vi "DrawGameOver.vi"(8 "error in (no error)":errorcluster, 11 "Game in":refnum<class "Game.lvclass">) -> (0 "error out":errorcluster, 3 "Game out":refnum<class "Game.lvclass">)   [LabVIEW 2019, in "RT_Game.lvlib" / "Game.lvclass"]
uses:
  Game.lvclass
  Color.ctl
  Coordinate.ctl
  Game.lvclass/Game.ctl
  RT_Game.lvlib
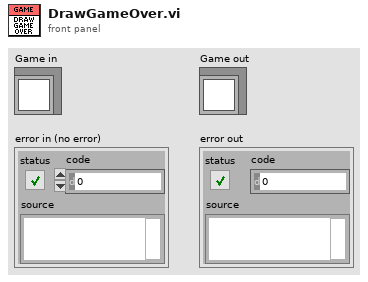
[diagram p1: front panel]
types:
  T1 = typedef "RT_Game.lvlib/Game.lvclass/Coordinate.ctl" = cluster{"x":dbl, "y":dbl}
  T2 = typedef "RT_Game.lvlib/Color.ctl" = fxp<+,3,3>
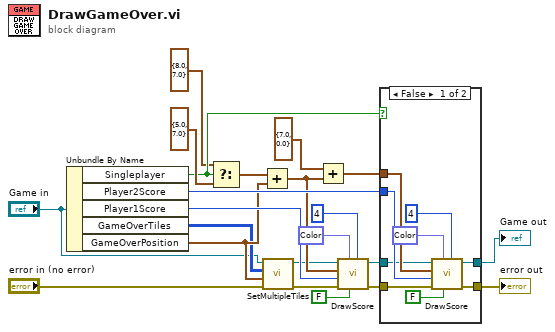
[diagram p0: block diagram]
diagram:
  n1 = Unbundle By Name("Game in") -> ("Singleplayer"=w2:bool, "Player2Score"=w22:i32, "Player1Score"=w14:i32, "GameOverTiles"=w7:u32[][], "GameOverPosition"=w12:T1)
  n2 = Select(t=T1 {"x"=8.0, "y"=7.0} ("f"), s=w2, f=T1 {"x"=5.0, "y"=7.0} ("x")) -> (s? t:f=w3:T1)
  n3 = Add(x=w3, y=w12) -> (x+y=w20:T1)
  n4 = call "SetMultipleTiles.vi"("error in (no error)"="error in (no error)", "Position"=w12, "TileCodes"=w7, "Game in"="Game in") -> ("error out"=w5:errorcluster, "Game out"=w9:refnum<class "Game.lvclass">)  [unwired: 6 in]
  n5 = Add(x=T1 {"x"=7.0, "y"=0.0}, y=w20) -> (x+y=w19:T1)
  n6 = call "DrawScore.vi"("Digits"=4, "AutoWidth?"=FALSE, "Color"=T2 1.0, "error in (no error)"=w5, "score"=w14, "position"=w20, "Pong in"=w9) -> ("error out"=w8:errorcluster, "Pong out"=w17:refnum<class "Game.lvclass">)  [unwired: 3 in]
  n7 = case shown="False" w2 {
    tunnel: w22 -> [w28 _]
    tunnel: w19 -> [w27 _]
    tunnel: [w26 w33] -> w18
    tunnel: w17 -> [w25 w33]
    tunnel: [w24 w32] -> w16
    tunnel: w8 -> [w23 w32]
    frame False {
      n8 = call "DrawScore.vi"("Digits"=4, "AutoWidth?"=FALSE, "Color"=T2 2.0, "error in (no error)"=w23, "score"=w28, "position"=w27, "Pong in"=w25) -> ("error out"=w24:errorcluster, "Pong out"=w26:refnum<class "Game.lvclass">)  [unwired: 3 in]
    }
    frame True {
    }
  }
  "Game out" <- w18
  "error out" <- w16
